vi "3HePressureCalculator.vi"(11 "Desired Tank\nPressure (3He)":dbl min=0.0 max=100.0 step=5.0) -> (0 "V2 Pressure (3He)":dbl min=0.0 max=100.0 step=5.0 format="%#.1f")   [LabVIEW 2018]
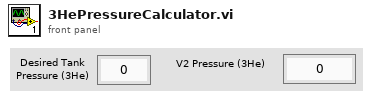
[diagram p1: front panel]
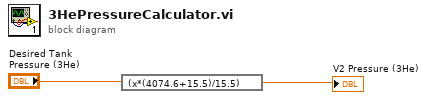
[diagram p0: block diagram]
diagram:
  n1 = expression code="(x*(4074.6+15.5)/15.5)"("Desired Tank\nPressure (3He)") -> (→"V2 Pressure (3He)":dbl)
